vi "MAIN_TL_wait_for_stabilization.vi"(0 "queue piezo":refnum<queue>, 1 "queue ASI stage":refnum<queue>, 2 "queue CAMERA":refnum<queue>, 3 "queue DAQ":refnum<queue>, 5 "DATA cluster":T1, 7 "Measure QPD":bool caption="Calibration", 9 "variant":variant, 11 "error in":errorcluster) -> (4 "Next task":T2, 15 "error out":errorcluster)   [LabVIEW 2015]
uses:
  CONTROLS/Q_main_element.ctl
  CONTROLS/Q_MCL_piezo_element.ctl
  CONTROLS/Q_ASI_stage_element.ctl
  CONTROLS/Q_DAQ_element.ctl
  CONTROLS/Q_camera_element.ctl
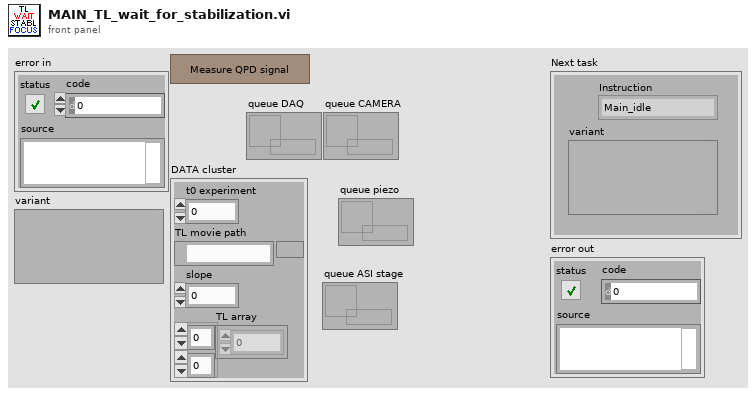
[diagram p1: front panel]
types:
  T1 = cluster{"t0 experiment":dbl, "TL movie path":path, "slope":dbl, "TL array":dbl[][]}
  T2 = typedef "Q_main_element.ctl" = cluster{"variant":variant, "Instruction":enum16{"Main_idle", "Main_initialize", "Main_initialize_TDMS", "Main_initialize_Queue", "Main_error", "Main_DAQ_initialization_results", "Main_ASI_initialization_results", "Main_Piezo_initialization_results", "Main_Valve_initialization_results", "Main_Pump_initialization_results", "Main_CAMERA_initialization_results", "Main_DAQ_error", "Main_ASI_error", "Main_Piezo_error", "Main_CAMERA_error", "Main_Valve_error", "Main_Pump_error", "Main_start_acquiring", "Main_not_acquiring", "Main_acquiring", "Main_stop_acquiring", "Main_change_exposure", "Main_change_z_scan_parameters", "Main_define_ROI", "Main_define_mosaic", "Main_read_kinetic_time", "Main_cooler", "Main_read_temperature", "Main_save_XY", "Main_load_XY", "Main_discard_XY", "Main_move_to_XY", "Main_measure_QPD", "Main_autofocus_calibration", "Main_save_PID", "Main_change_H_valve_position", "Main_two_way_valve", "Main_save_movie", "Main_init_single_scan", "Main_single_scan", "Main_stop_single_scan", "Main_merFISH_illumination_parameters", "Main_merFISH_buffer_probe_list", "Main_merFISH_injections_procedure", "Main_merFISH_save_setpoint", "Main_merFISH_DAPI_parameters", "Main_merFISH_Brightfield_parameters", "Main_merFISH_save_embryo_ROI", "Main_merFISH_init", "Main_merFISH_resume", "Main_merFISH_start_autofocus", "Main_merFISH_open_close_valve_merFISH", "Main_merFISH_open_close_valve_photobleaching", "Main_merFISH_hybridization", "Main_merFISH_move_to_ROI", "Main_merFISH_wait_stabilization", "Main_merFISH_scan_laser", "Main_merFISH_scan_brightfield", "Main_merFISH_photobleaching_injection", "Main_merFISH_photobleaching", "Main_merFISH_save", "Main_merFISH_send_email", "Main_merFISH_close", "Main_TL_define_parameters", "Main_TL_reset_parameters", "Main_TL_init", "Main_TL_start_autofocus", "Main_TL_move_to_ROI", "Main_TL_wait_for_stabilization", "Main_TL_scan", "Main_TL_wait_cycle_end", "Main_TL_close", "Main_STOP"}}
  T3 = cluster{"i":i32, "data":cluster{"Channel":string, "ROI #":i32}}
  T4 = cluster{"Measure QPD":bool, "data":cluster{"Channel":string, "ROI #":i32}, "t0 experiment":dbl, "TL movie path":path, "slope":dbl, "QPD setpoint":cluster{"X":dbl, "Y":dbl, "intensity":dbl}, "N Frames":i32}
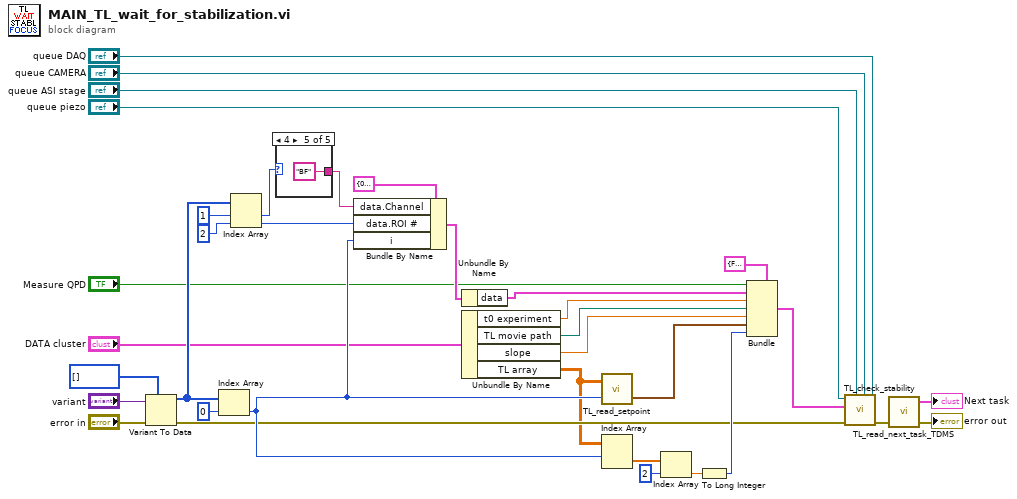
[diagram p0: block diagram]
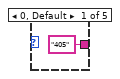
[diagram p2: hidden frame]
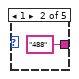
[diagram p3: hidden frame]
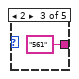
[diagram p4: hidden frame]
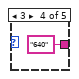
[diagram p5: hidden frame]
diagram:
  n1 = Variant To Data(error in="error in", type=i32[] [] ("appended array"), Variant="variant") -> (data=w26:i32[], error out=w15:errorcluster)
  n2 = Index Array(array=w26, index=0) -> (element=w33:i32)
  n3 = Index Array(array=w26, index #1=1 ("index"), index #2=2 ("index")) -> (element #1=w30:i32, element #2=w32:i32)
  n4 = case shown="4" w30 {
    tunnel: ["405" "488" "561" "640" "BF"] -> w31
    frame 0, Default {
    }
    frame 1 {
    }
    frame 2 {
    }
    frame 3 {
    }
    frame 4 {
    }
  }
  n5 = Bundle By Name(cluster=T3 {"i"=0, "data"={"Channel"="", "ROI #"=0}} ("output cluster"), "data.Channel"=w31, "data.ROI #"=w32, "i"=w33) -> (w34:T3)
  n6 = Unbundle By Name(w34) -> ("data"=w20:cluster{"Channel":string, "ROI #":i32})
  n7 = Unbundle By Name("DATA cluster") -> ("t0 experiment"=w21:dbl, "TL movie path"=w16:path, "slope"=w17:dbl, "TL array"=w14:dbl[][])
  n8 = call "TL_read_setpoint.vi"("setpoint #"=w33, "TL array"=w14) -> ("QPD setpoint"=w18:cluster{"X":dbl, "Y":dbl, "intensity":dbl})  [unwired: 1 in]
  n9 = Index Array(array=w14, index (row)=w33) -> (element=w13:dbl[])  [unwired: 1 in]
  n10 = Index Array(array=w13, index=2) -> (element=w11:dbl)
  n11 = To Long Integer(number=w11) -> (32bit integer=w19:i32)
  n12 = Bundle(cluster=T4 {"Measure QPD"=FALSE, "data"={"Channel"="", "ROI #"=0}, "t0 experiment"=0.0, "TL movie path"=path "", "slope"=0.0, "QPD setpoint"={"X"=0.0, "Y"=0.0, "intensity"=0.0}, "N Frames"=0} ("output cluster"), "Measure QPD"="Measure QPD", "data"=w20, "t0 experiment"=w21, "TL movie path"=w16, "slope"=w17, "QPD setpoint"=w18, "N Frames"=w19) -> (w23:T4)
  n13 = call "TL_check_stability.vi"("queue DAQ"="queue DAQ", "queue CAMERA"="queue CAMERA", "queue ASI stage"="queue ASI stage", "error in"=w15, "Data cluster"=w23, "queue piezo"="queue piezo") -> ("error out"=w35:errorcluster)  [unwired: 5 in]
  n14 = call "TL_read_next_task_TDMS.vi"("error in"=w35) -> ("error out"=→"error out":errorcluster, "task"=→"Next task":T2)  [unwired: 3 in]
